vi "SetUpDigitalOutput.vi"(8 "error in (no error)":errorcluster, 11 "TesteractHAL_DigitalOutput_NIDAQmx In":refnum<class "TesteractHAL_DigitalOutput_NIDAQmx.lvclass">) -> (0 "error out":errorcluster, 3 "TesteractHAL_DigitalOutput_NIDAQmx Out":refnum<class "TesteractHAL_DigitalOutput_NIDAQmx.lvclass">)   [LabVIEW 2017, in "TesteractHAL_DigitalOutput_NIDAQmx.lvlib" / "TesteractHAL_DigitalOutput_NIDAQmx.lvclass"]
doc: "Sets up the device as a DAQmx digital output."
uses:
  TesteractHAL_DigitalOutput_NIDAQmx.lvclass
  TesteractHAL_DigitalOutput_NIDAQmx.lvclass/TesteractHAL_DigitalOutput_NIDAQmx.ctl
  <vilib>/DAQmx/create/channels.llb/DAQmx Create Channel (DO-Digital Output).vi
  <resource>/objmgr/daqmx.rc
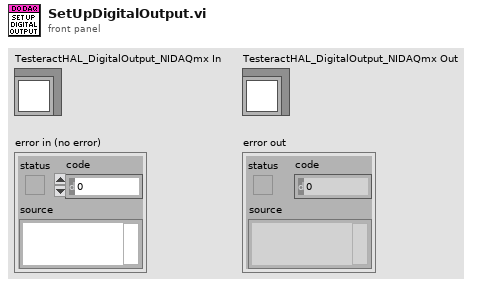
[diagram p1: front panel]
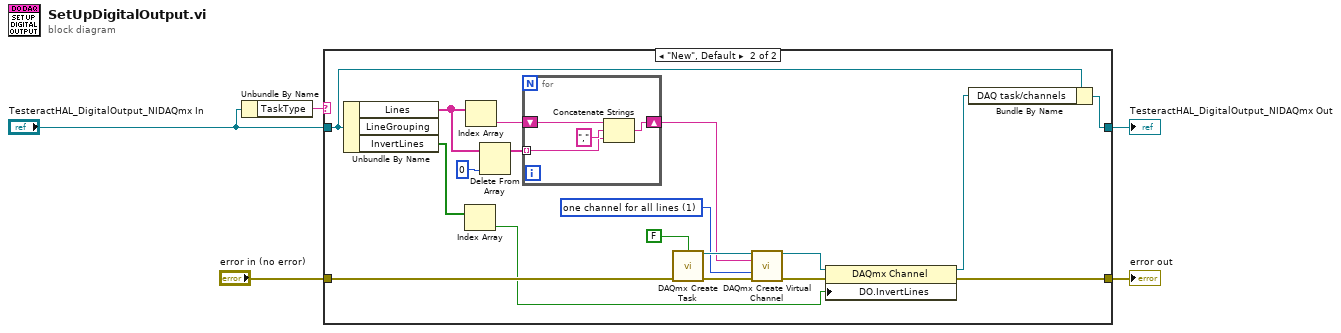
[diagram p0: block diagram]
diagram:
  n1 = Unbundle By Name("TesteractHAL_DigitalOutput_NIDAQmx In") -> ("TaskType"=w1:string)
  n2 = case shown="\"New\", Default" w1 {
    tunnel: "error in (no error)" -> [w6 w23]
    tunnel: [w6 w21] -> w4
    tunnel: [w7 w20] -> w3
    tunnel: "TesteractHAL_DigitalOutput_NIDAQmx In" -> [w7 w19]
    frame "Existing" {
      # "Fill this in when it's needed!!!!!\nThis is for tasks that are already set up in MAX"
    }
    frame "New", Default {
      w8 = 1 items=["one channel for each line", "one channel for all lines"] ("line grouping")
      n3 = Unbundle By Name(w19) -> ("Lines"=w12:string[], "InvertLines"=w10:bool[])  [unwired: 1 out]
      n4 = Index Array(array=w10) -> (element=w9:bool)  [unwired: 1 in]
      n5 = Index Array(array=w12) -> (element=w14:string)  [unwired: 1 in]
      n6 = Delete From Array(array=w12, index=0) -> (array with subset deleted=w13:string[])  [unwired: 1 in, 1 out]
      n7 = for {
        shift-right: [w28] -> w11
        shift-left: w14 -> [w27]
        tunnel: w13 -> [w26] mode=indexing
        n8 = Concatenate Strings(w27, ",", w26) -> (w28:string)
      }
      n9 = call <vilib>:"DAQmx Create Task.vi"("auto cleanup"=FALSE, "error in"=w23) -> ("task out"=w24:refnum<k21>, "error out"=w25:errorcluster)  [unwired: 12 in]
      n10 = call-poly <vilib>:"DAQmx Create Virtual Channel.vi"("task in"=w24, "lines"=w11, "line grouping"=w8, "error in"=w25) -> ("task out"=w16:refnum<k21>, "error out"=w17:errorcluster)  [unwired: 10 in]
      n11 = property class="DAQmx Channel"(reference=w16, error in=w17, "DO.InvertLines"=w9) -> (reference out=w22:refnum<k21>, error out=w21:errorcluster)
      n12 = Bundle By Name(cluster=w19, "DAQ task/channels"=w22) -> (w20:refnum<class "TesteractHAL_DigitalOutput_NIDAQmx.lvclass">)
    }
  }
  "error out" <- w4
  "TesteractHAL_DigitalOutput_NIDAQmx Out" <- w3
